vi "Choreo_TrajectoryCacheSwerve_LoadTrajectory.vi"(11 "TrajectoryName":string) -> (0 "error out":errorcluster, 3 "ChoreoTrajectorySwerve":T1)   [LabVIEW 2019, in "ChoreoLib.lvlib"]
doc: "Load a Choreo trajectory from a JSON formatted file. Note that for newer versions of Choreo, the file has a \".traj\" extension. Internally this is formatted as a JSON file.\n\nInputs: \n - filename - string - The name of the trajectory file. See notes below on file naming.\n\nOutputs:\n - Trajectory - cluster - Trajectory read from JSON file.\n - Error out - cluster - Error cluster\n - Full Filename - string - fully qualified file name.\n\nNotes on file naming:\n - The file name must include the extention. \".json\", or \".traj\" is not automatically appended to the name. \n - The file name can be a simple file or an absolute path. If a simple file name is used the default path on the RoboRIO is: \"home:\\lvuser\\natinst\\LabVIEW Data\". On a Windows PC the default path is the LabVIEW default directory. Normally this is: “%HOMEDRIVE%%HOMEPATH%\\Documents\\LabView Data\".\n - Filenames on the RoboRIO, which runs Linux, are case sensitive."
uses:
  ChoreoLib.lvlib
  Choreo_ChoreoSwerve_Globals.vi
  TypeDef/ChoreoSwerveSample.ctl
  TypeDef/ChoreoEventMarker.ctl
  TypeDef/ChoreoTrajectorySwerve.ctl
panel:
  in  "error in (no error)":errorcluster
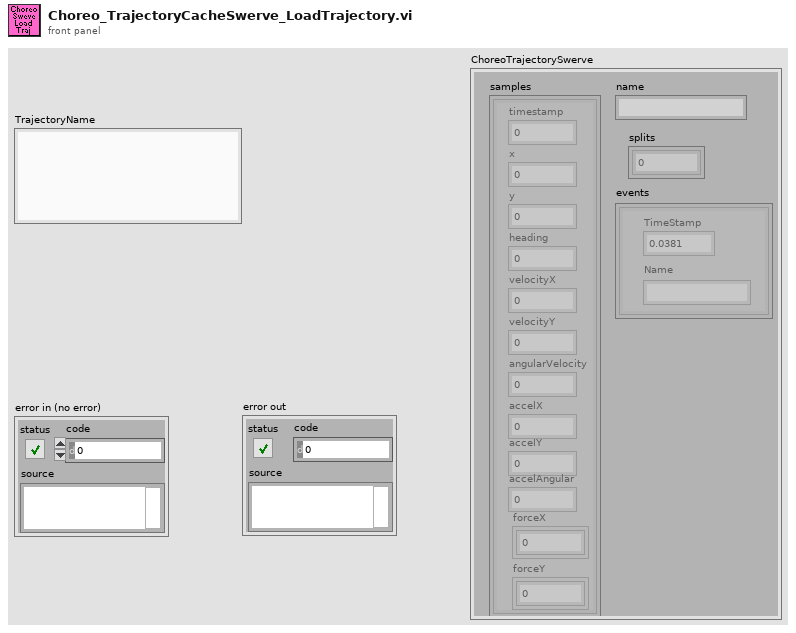
[diagram p1: front panel]
types:
  T1 = typedef "ChoreoLib.lvlib/ChoreoTrajectorySwerve.ctl" = cluster{"name":string, "samples":T2[], "splits":i32[], "events":T3[]}
  T2 = typedef "ChoreoLib.lvlib/ChoreoSwerveSample.ctl" = cluster{"timestamp":dbl, "x":dbl, "y":dbl, "heading":dbl, "velocityX":dbl, "velocityY":dbl, "angularVelocity":dbl, "accelX":dbl, "accelY":dbl, "accelAngular":dbl, "forceX":dbl[], "forceY":dbl[]}
  T3 = typedef "ChoreoLib.lvlib/ChoreoEventMarker.ctl" = cluster{"TimeStamp":dbl, "Name":string}
  T4 = typedef "ChoreoLib.lvlib/ChoreoTrajectoryCacheSwerve.ctl" = map{string, T1}
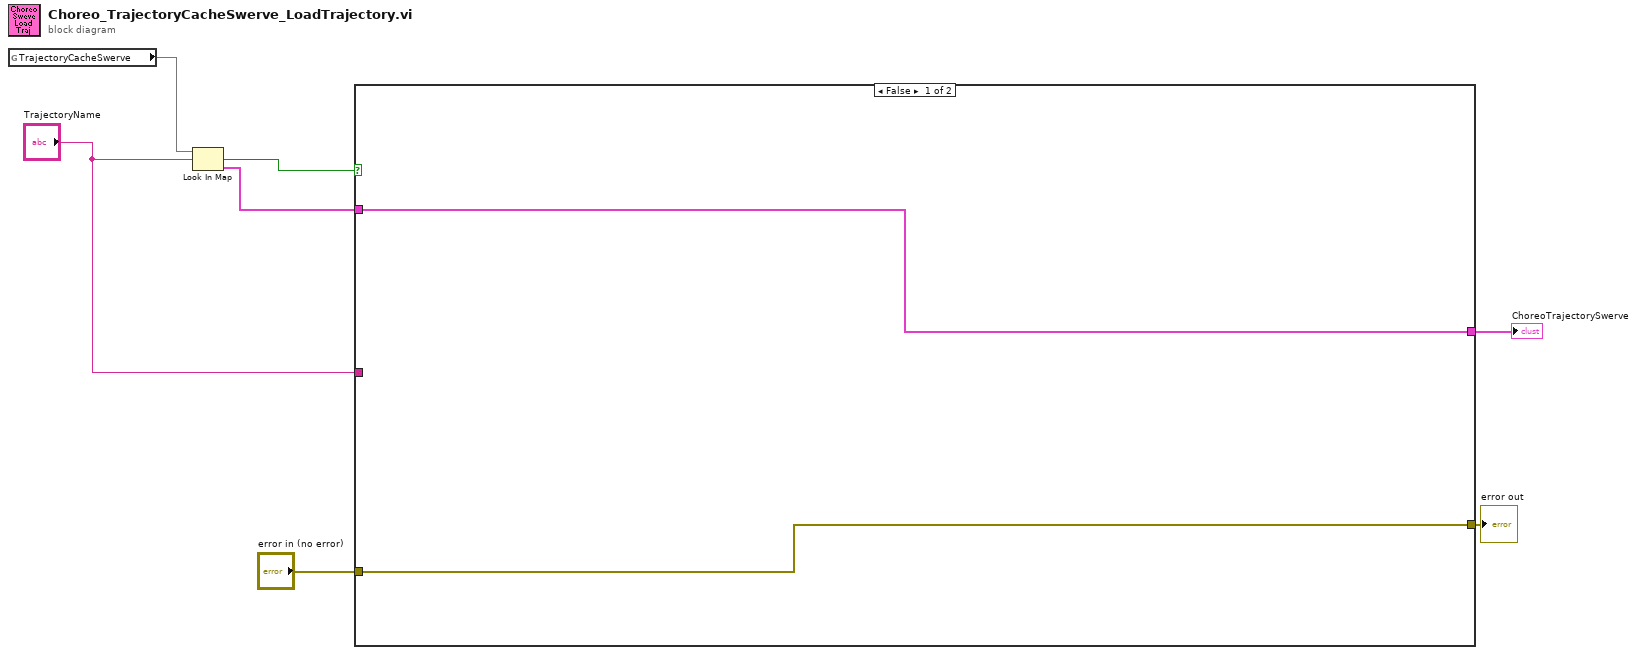
[diagram p0: block diagram]
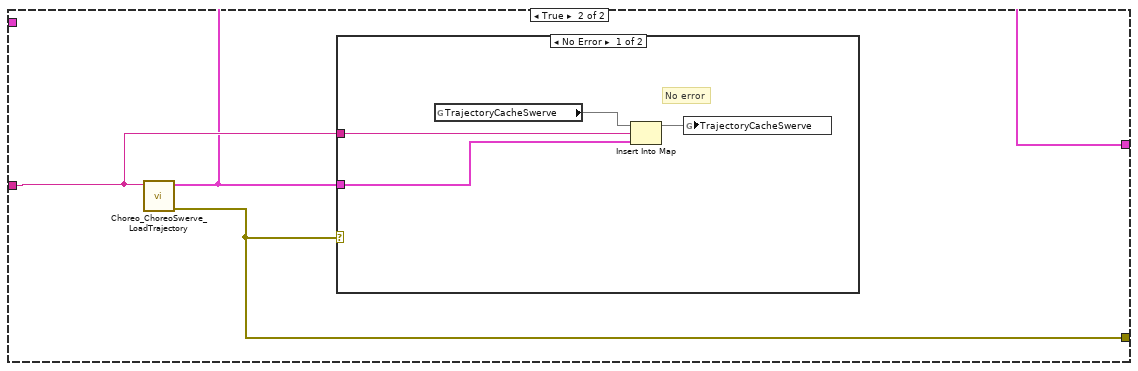
[diagram p2: hidden frame]
diagram:
  n1 = global read "Choreo_ChoreoSwerve_Globals.vi" "TrajectoryCacheSwerve"() -> (w4:T4)
  n2 = Look In Map(map=w4, key="TrajectoryName") -> (key not found?=w2:bool, value=w1:T1)  [unwired: 1 in]
  n3 = case shown="False" w2 {
    tunnel: "error in (no error)" -> [w8 _]
    tunnel: [w8 w12] -> w6
    tunnel: [w9 w10] -> w5
    tunnel: "TrajectoryName" -> [_ w11]
    tunnel: w1 -> [w9 _]
    frame False {
    }
    frame True {
      n4 = call "Choreo_ChoreoSwerve_LoadTrajectory.vi"("FileName"=w11) -> ("error out"=w12:errorcluster, "ChoreoTrajectorySwerve"=w10:T1)  [unwired: 8 in, 1 out]
      n5 = case shown="No Error" w12 {
        tunnel: w11 -> [w14 _]
        tunnel: w10 -> [w13 _]
        frame No Error {
          # "No error"
          n6 = global read "Choreo_ChoreoSwerve_Globals.vi" "TrajectoryCacheSwerve"() -> (w16:T4)
          n7 = Insert Into Map(map in=w16, key=w14, value=w13) -> (map out=w15:T4)  [unwired: 2 out]
          n8 = global write "Choreo_ChoreoSwerve_Globals.vi" "TrajectoryCacheSwerve"(w15) -> ()
        }
        frame Error {
        }
      }
    }
  }
  "error out" <- w6
  "ChoreoTrajectorySwerve" <- w5
